vi "m10.wfg.03PT.vi"(1 "Param 0":dbl, 2 "Param 1":dbl, 3 "Param 2":dbl, 4 "Param 3":dbl, 5 "error in (no error)":errorcluster, 8 "Waveform Properties":T1 {"Ramp (s)" min=0.0; "Fs (Hz)" min=0.0}) -> (14 "Waveform Out":waveform(dbl), 19 "error out":errorcluster)   [LabVIEW 2009]
uses:
  <vilib>/measure/NI_MABase.lvlib
panel:
  # "Pure Tone Frequency"
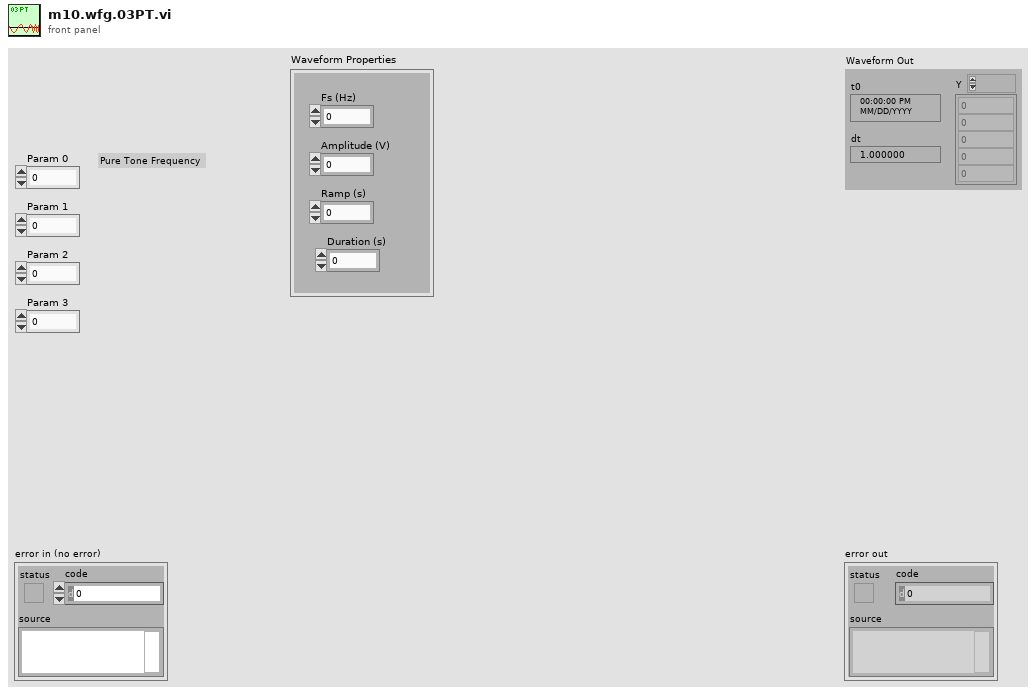
[diagram p1: front panel]
types:
  T1 = cluster{"Fs (Hz)":dbl, "Amplitude (V)":dbl, "Ramp (s)":dbl, "Duration (s)":dbl}
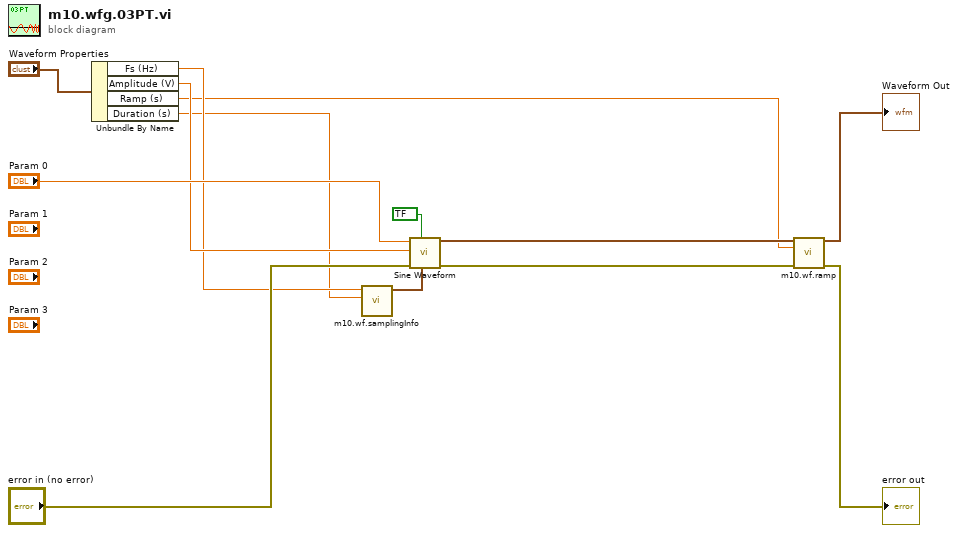
[diagram p0: block diagram]
diagram:
  n1 = Unbundle By Name("Waveform Properties") -> ("Fs (Hz)"=w7:dbl, "Amplitude (V)"=w10:dbl, "Ramp (s)"=w4:dbl, "Duration (s)"=w1:dbl)
  n2 = call "m10.wf.samplingInfo.vi"("Duration (s)"=w1, "Fs (Hz)"=w7) -> ("sampling info"=w8:cluster{"Fs":dbl, "#s":dbl})  [unwired: 9 in]
  n3 = call <vilib>:"Sine Waveform.vi"("sampling info"=w8, "reset signal"=bool ?, "error in (no error)"="error in (no error)", "amplitude"=w10, "frequency"="Param 0") -> ("error out"=w3:errorcluster, "signal out"=w5:waveform(dbl))  [unwired: 5 in]
  n4 = call "m10.wf.ramp.vi"("Waveform In"=w5, "Ramp Length (s)"=w4, "error in (no error)"=w3) -> ("Waveform Out"=→"Waveform Out":waveform(dbl), "error out"=→"error out":errorcluster)  [unwired: 11 in]
